vi "ReadTSV.vi"(11 "Path":path) -> (2 "Complex FRF":cluster{dbl, "df":dbl, cdb[]}, 3 "all rows":dbl[][](array[numeric]))   [LabVIEW 2022 SP3]
uses:
  Mic/Mic_Global.vi
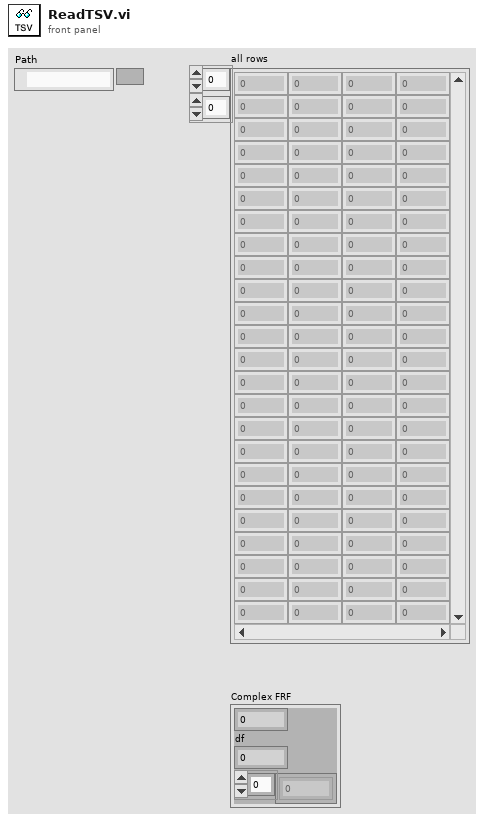
[diagram p1: front panel]
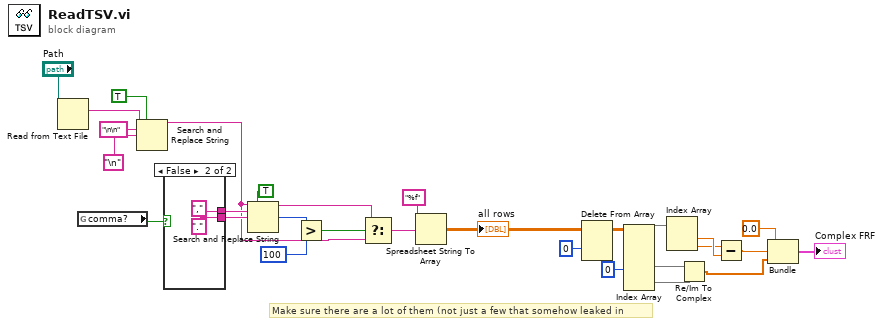
[diagram p0: block diagram]
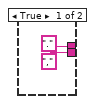
[diagram p2: hidden frame]
diagram:
  # "Make sure there are a lot of them (not just a few that somehow leaked in"
  n1 = Read from Text File(file (use dialog)="Path") -> (text=w12:string)  [unwired: 3 in, 3 out]
  n2 = global read "Mic_Global.vi" "comma?"() -> (w8:bool)
  n3 = Search and Replace String(replace all?=TRUE ("replace all? (F)"), input string=w12, search string="\n\n", replace string="\n" ("search string")) -> (result string=w2:string)  [unwired: 4 in, 3 out]
  n4 = case shown="False" w8 {
    tunnel: ["." ("search string") "," ("search string")] -> w10
    tunnel: ["," ("search string") "." ("search string")] -> w7
    frame True {
    }
    frame False {
    }
  }
  n5 = Search and Replace String(replace all?=TRUE ("replace all? (F)"), input string=w2, search string=w10, replace string=w7) -> (result string=w3:string, number of replacements=w6:i32)  [unwired: 4 in, 2 out]
  n6 = Greater?(x=w6, y=100) -> (0:w4:bool)
  n7 = Select(t=w3, s=w4, f=w2) -> (s? t:f=w1:string)
  n8 = Spreadsheet String To Array(format string="%f", spreadsheet string=w1) -> (array=w17:dbl[][])  [unwired: 2 in]
  "all rows" <- w17
  n9 = Delete From Array(array=w17, index (row)=0) -> (array with subset deleted=w19:dbl[][])  [unwired: 2 in, 1 out]
  n10 = Index Array(array=w19, index (col) #1=0 ("disabled index (col)")) -> (element #1=w20:dbl[], element #2=w28:dbl[], element #3=w29:dbl[])  [unwired: 5 in]
  n11 = Index Array(array=w20) -> (element #1=w22:dbl, element #2=w21:dbl)  [unwired: 2 in]
  n12 = Re/Im To Complex(1:w29, 2:w28) -> (0:w25:cdb[])
  n13 = Subtract(x=w21, y=w22) -> (x-y=w23:dbl)
  n14 = Bundle(0.0, w23, w25) -> (→"Complex FRF":cluster{dbl, dbl, cdb[]})  [unwired: 1 in]
